vi "State History.vi"(4 "Max History\nLength (50)":i32=50, 6 "Reset?":bool, 7 "History Name":string, 10 "State In":string) -> ()   [LabVIEW 2013, in "State Machine Lib.lvlib"]
doc: "Reentrant VI. Place this after the pop state in the queued state machine for debugging stateQ tracing"
uses:
  State Machine Lib.lvlib
panel:
  out "History":T1(array[cluster])
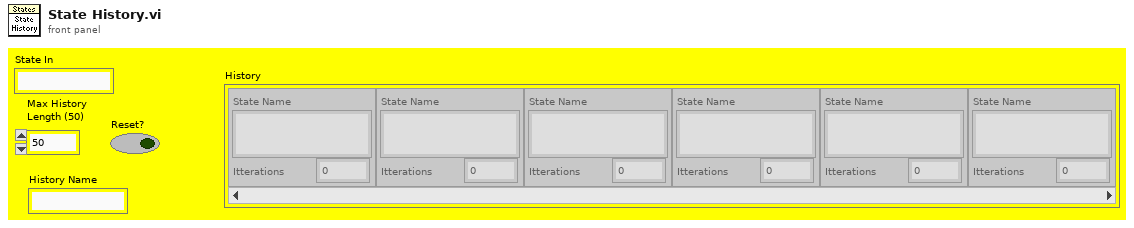
[diagram p1: front panel]
types:
  T1 = cluster{"State Name":string, "Itterations":u32}[]
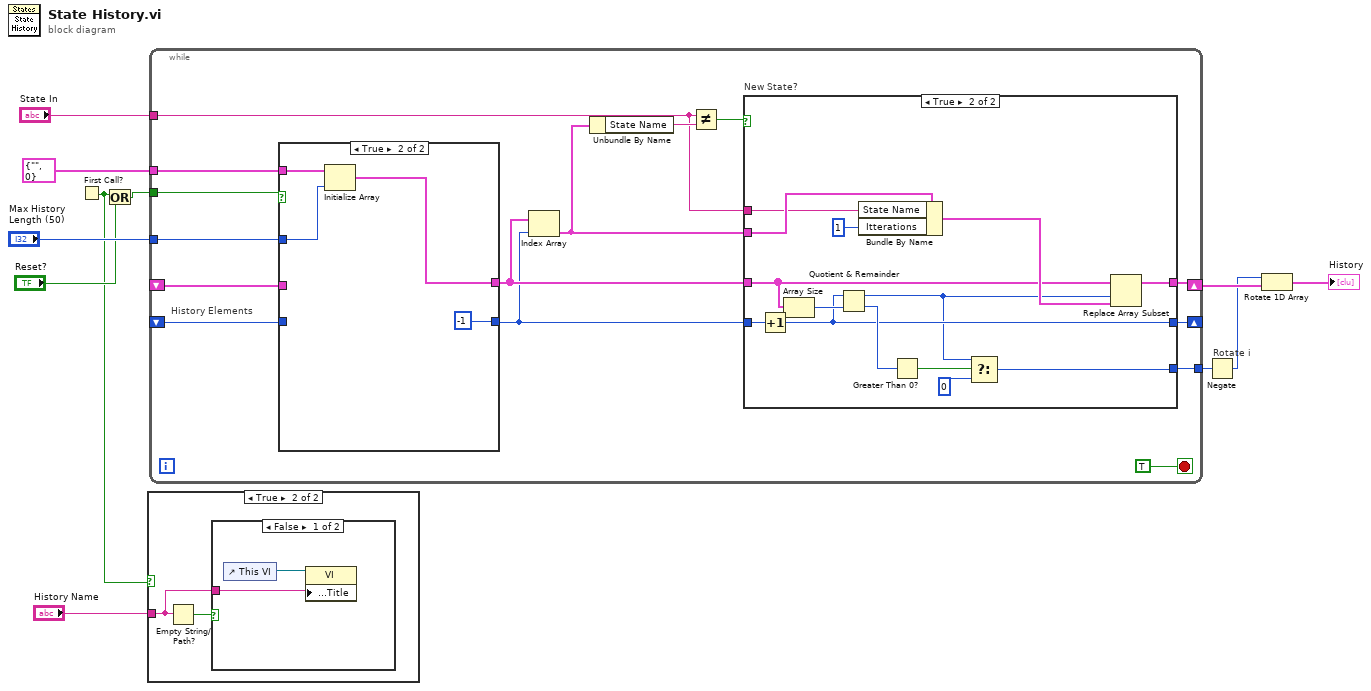
[diagram p0: block diagram]
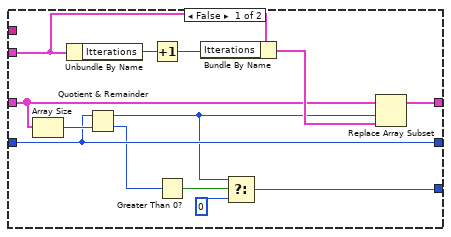
[diagram p4: hidden frame]
diagram:
  # "Rotate i"
  n1 = First Call?() -> (First Call?: T/F=w2:bool)
  n2 = Or(x=w2, y="Reset?") -> (x .or. y?=w4:bool)
  n3 = case shown="True" w2 {
    tunnel: "History Name" -> [_ w12]
    frame False {
    }
    frame True {
      n4 = Empty String/Path?(string/path=w12) -> (empty?=w13:bool)
      n5 = case shown="False" w13 {
        tunnel: w12 -> [w14 _]
        frame False {
          n6 = control-ref of="This VI"() -> (w15:refnum<vi>)
          n7 = property class="VI"(reference=w15, "Front Panel.Title"=w14) -> ()  [unwired: 1 in, 2 out]
        }
        frame True {
        }
      }
    }
  }
  n8 = while {
    shift-right: [w24] -> w8
    shift-left: _ -> [w26]
    tunnel: w4 -> [w29]
    tunnel: "Max History\nLength (50)" -> [w28]
    tunnel: cluster{"State Name":string, "Itterations":u32} {"State Name"="", "Itterations"=0} ("History Element") -> [w27]
    shift-right: [w17] -> _
    shift-left: _ -> [w25]
    tunnel: "State In" -> [w20]
    tunnel: [w16] -> w7
    stop <- TRUE stop-if-true
    # "History Elements"
    n9 = case shown="True" w29 {
      tunnel: w28 -> [_ w62]
      tunnel: w27 -> [_ w63]
      tunnel: [w59 -1 ("Max History Length")] -> w18
      tunnel: w26 -> [w58 _]
      tunnel: w25 -> [w59 _]
      tunnel: [w58 w60] -> w19
      frame False {
      }
      frame True {
        n10 = Initialize Array(w63, w62) -> (w60:T1)
      }
    }
    n11 = Index Array(array=w19, index=w18) -> (element=w23:cluster{"State Name":string, "Itterations":u32})
    n12 = Unbundle By Name(w23) -> ("State Name"=w22:string)
    n13 = Not Equal?(x=w20, y=w22) -> (x != y?=w21:bool)
    n14 = case "New State?" shown="True" w21 {
      tunnel: w19 -> [w37 w53]
      tunnel: [w43 w57] -> w24
      tunnel: w23 -> [w40 w56]
      tunnel: w20 -> [_ w50]
      tunnel: w18 -> [w36 w52]
      tunnel: [w36 w49] -> w17
      tunnel: [w32 w44] -> w16
      frame False {
        n15 = Array Size(array=w37) -> (size(s)=w38:i32)
        n16 = Unbundle By Name(w40) -> ("Itterations"=w42:u32)
        n17 = Quotient & Remainder(x=w36, y=w38) -> (x-y*floor(x/y)=w31:i32, floor(x/y)=w35:i32)
        n18 = Increment(x=w42) -> (x+1=w41:u32)
        n19 = Greater Than 0?(x=w35) -> (x > 0?=w34:bool)
        n20 = Bundle By Name(cluster=w40, "Itterations"=w41) -> (w39:cluster{"State Name":string, "Itterations":u32})
        n21 = Select(t=w31, s=w34, f=0 ("floor(x/y)")) -> (s? t:f=w32:i32)
        n22 = Replace Array Subset(array=w37, new element=w39, index=w31) -> (w43:T1)
      }
      frame True {
        n23 = Increment(x=w52) -> (x+1=w49:i32)
        n24 = Array Size(array=w53) -> (size(s)=w54:i32)
        n25 = Quotient & Remainder(x=w49, y=w54) -> (x-y*floor(x/y)=w45:i32, floor(x/y)=w51:i32)
        n26 = Bundle By Name(cluster=w56, "State Name"=w50, "Itterations"=u32 1) -> (w55:cluster{"State Name":string, "Itterations":u32})
        n27 = Greater Than 0?(x=w51) -> (x > 0?=w46:bool)
        n28 = Select(t=w45, s=w46, f=0 ("floor(x/y)")) -> (s? t:f=w44:i32)
        n29 = Replace Array Subset(array=w53, new element=w55, index=w45) -> (w57:T1)
      }
    }
  }
  n30 = Negate(x=w7) -> (-x=w6:i32)
  n31 = Rotate 1D Array(1:w8, 2:w6) -> (0:→"History":T1)
